vi "多影像平均_二值化_抓邊 _圓ROI.vi"() -> ()   [LabVIEW 2015]
uses:
  <vilib>/vision/Measure.llb/Edge Options.ctl
  <vilib>/vision/Measure.llb/Edge Polarity.ctl
  <vilib>/userdefined/High Color/IMAQdx.ctl
  <vilib>/Utility/miscctls.llb/LVPositionTypeDef.ctl
  <vilib>/Analysis/coordinate.llb/2D Cartesian Coordinate Rotation (Scalar).vi
  <vilib>/vision/NI_Vision_Development_Module.lvlib
  <vilib>/vision/driver/NI_Vision_Acquisition_Software.lvlib
  <resource>/objmgr/imaqdx.rc
  <vilib>/Analysis/NI_AALPro.lvlib
panel:
  in  "處理平均影像":bool
  out "Ellipse":T1 {"Minor Axis"."Point 2"."Y" format="%.2f"; "Minor Axis"."Point 2"."X" format="%.2f"; "Minor Axis"."Point 1"."Y" format="%.2f"; "Minor Axis"."Point 1"."X" format="%.2f"; "Major Axis"."Point 2"."Y" format="%.2f"; "Major Axis"."Point 2"."X" format="%.2f"; "Major Axis"."Point 1"."Y" format="%.2f"; "Major Axis"."Point 1"."X" format="%.2f"; "Center"."Y" format="%.2f"; "Center"."X" format="%.2f"}
  in  "載入影像":bool
  in  "拍攝影像":bool
  in  "影像數量":i32=4
  out "二值化影像陣列":T2[](array[plugin-control])
  out "全部影像Histograph":T3(graph)
  out "Image binary":T2(plugin-control)
  out "平均影像Histograph":T4(graph)
  out "Standard Deviation":sgl format="%#.2f"
  out "Mean":sgl format="%#.2f"
  out "影像陣列":T2[](array[plugin-control])
  in  "stop":bool
  in  "Horizontal Progress Bar":u8(slide) scale=0.0..255.0
  out "Image mean":T2(plugin-control)
  out "取像編號":i32
  out "取像視窗":T2(plugin-control)
  in  "Session In":T5="cam1"
  out "degrees":sgl
  in  "Edge Options":T6={"Edge Polarity"=0, "Kernel Size"=3, "Width"=3, "Minimum Edge Strength"=10.0, "Interpolation Type"=enum."Bilinear Fixed", "Data Processing Method"=enum."Average"} {"Edge Polarity" items=["All Edges", "Rising Edges", "Falling Edges"]; "Minimum Edge Strength" format="%.2f"; "Width" step=2; "Kernel Size" step=2}
  out "Gradient Information":dbl[][](graph)
  out "Line Segment":T8 {"Point 2"."Y" format="%.2f"; "Point 2"."X" format="%.2f"; "Point 1"."Y" format="%.2f"; "Point 1"."X" format="%.2f"}
  out "error out":errorcluster
  in  "Direction":T9(ring)
  in  "Process":T10(ring)
  out "Line Profile":T11(graph)
  in  "Gap":i32=10 min=1 max=300
  out "Image":T2(plugin-control)
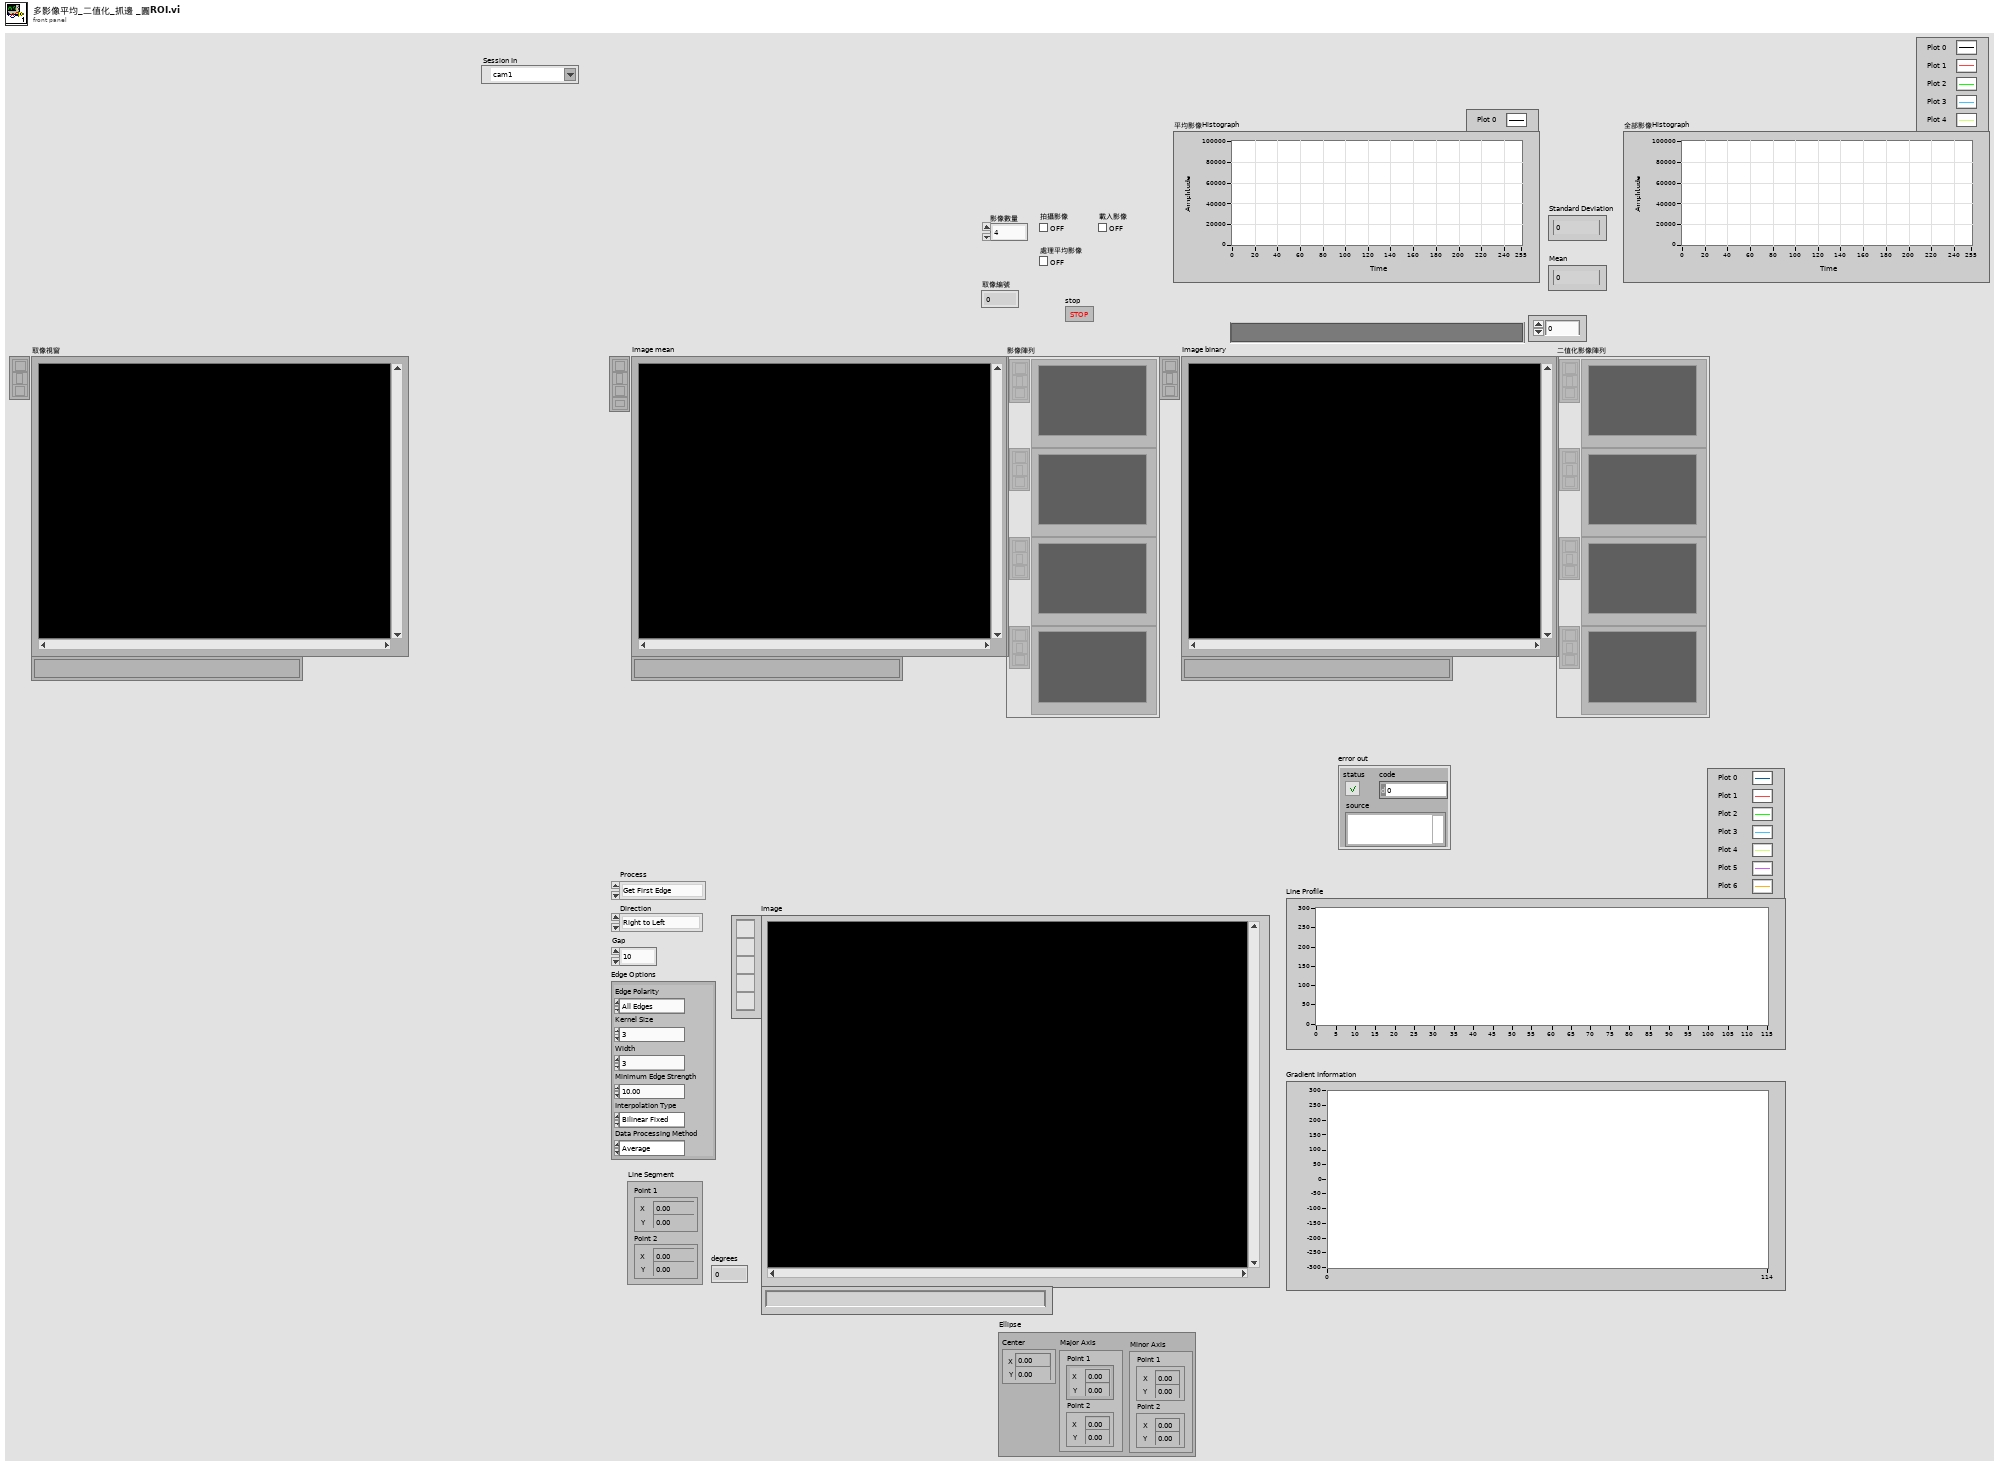
[diagram p1: front panel]
types:
  T1 = cluster{"Center":cluster{"X":sgl, "Y":sgl}, "Major Axis":cluster{"Point 1":cluster{"X":sgl, "Y":sgl}, "Point 2":cluster{"X":sgl, "Y":sgl}}, "Minor Axis":cluster{"Point 1":cluster{"X":sgl, "Y":sgl}, "Point 2":cluster{"X":sgl, "Y":sgl}}}
  T2 = typedef "IMAQ Image.ctl" = refnum<image>
  T3 = cluster{"Starting Value":sgl, "Incremental Value":sgl, "Histogram":u32[]}[]
  T4 = cluster{"Starting Value":sgl, "Incremental Value":sgl, "Histogram":u32[]}
  T5 = typedef "IMAQdx.ctl" = refnum<k21>
  T6 = typedef "Edge Options.ctl" = cluster{"Edge Polarity":T7, "Kernel Size":u32, "Width":u32, "Minimum Edge Strength":sgl, "Interpolation Type":enum32{"Zero Order", "Bilinear", "Quadratic", "Cubic", "Bilinear Fixed"}, "Data Processing Method":enum32{"Average", "Median"}}
  T7 = typedef "Edge Polarity.ctl" = u32
  T8 = cluster{"Point 1":cluster{"X":sgl, "Y":sgl}, "Point 2":cluster{"X":sgl, "Y":sgl}}
  T9 = enum16{"Right to Left", "Left  to Right", "Up to Down", "Down to Up", "Inner to Outer", "Outer to Inner"}
  T10 = enum16{"Get First Edge", "Get First + Last Edge", "Get All Edges", "Get Best Edge"}
  T11 = cluster{"x0":sgl, "dx":sgl, "Pixels Line":sgl[]}[]
  T12 = typedef "LVPositionTypeDef.ctl" = cluster{"Left":i32, "Top":i32}
  T13 = typedef "Image Type" = u32
  T14 = cluster{"Global Rectangle":i32[], "Contours":cluster{"Contour Type":u32, "ROI Type":u32, "Points":i32[]}[]}
  T15 = typedef "IMAQ Rectangle" = cluster{"Left":i32, "Top":i32, "Right":i32, "Bottom":i32, "Rotation":dbl}
  T16 = typedef "IMAQ Point" = cluster{"X":sgl, "Y":sgl}
  T17 = typedef "IMAQ Circle" = cluster{"Center X":i32, "Center Y":i32, "Inner Radius":i32, "Outer Radius":i32, "Start Angle":dbl, "End Angle":dbl}
  T18 = cluster{"Point 1":cluster{"x":dbl, "y":dbl}, "Point 2":cluster{"x":dbl, "y":dbl}}
  T19 = typedef "IMAQ Line" = cluster{"Start X":i32, "Start Y":i32, "End X":i32, "End Y":i32}
  T20 = cluster{"Contour Type":u32, "ROI Type":u32, "Points":i32[]}[]
  T21 = cluster{"Contour Type":u32, "ROI Type":u32, "Points":i32[]}
  T22 = typedef "ROI Descriptor" = cluster{"Global Rectangle":i32[], "Contours":cluster{"ID":enum32{"External", "Internal"}, "Type":u32, "Coordinates":i32[]}[]}
  T23 = typedef "Edge New.ctl" = cluster{"Location (Pixel)":cluster{"X":sgl, "Y":sgl}, "Location (Real-World)":cluster{"X":sgl, "Y":sgl}, "Distance (Pixel)":dbl, "Distance (Real-World)":dbl, "Strength":dbl, "Noise":dbl, "Rising?":bool}
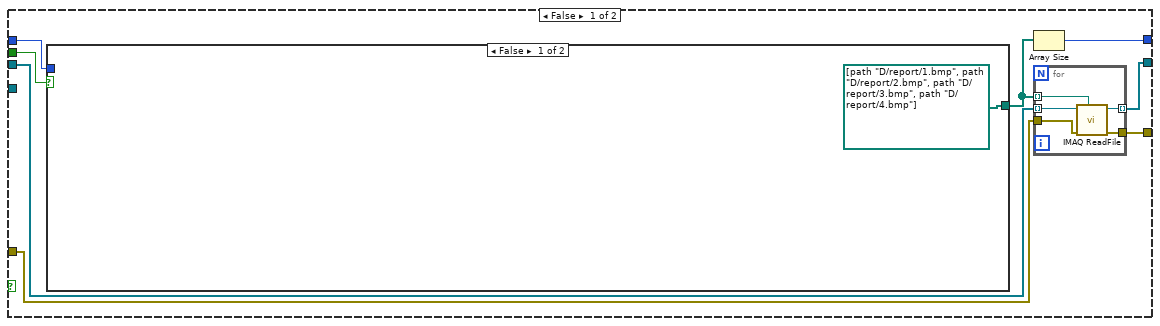
[diagram p2: hidden frame]
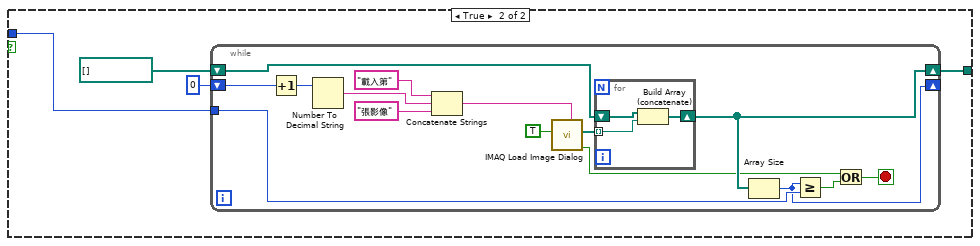
[diagram p3: hidden frame]
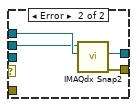
[diagram p4: hidden frame]
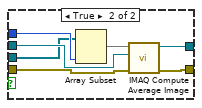
[diagram p5: hidden frame]
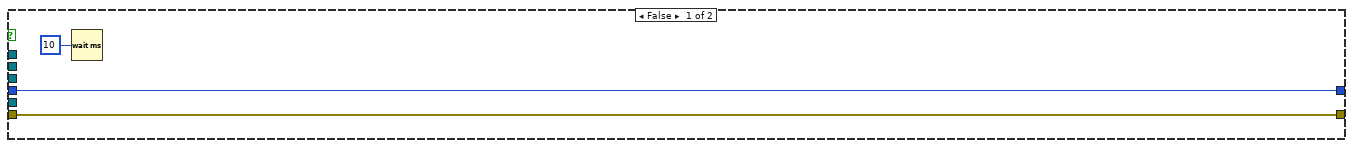
[diagram p6: hidden frame]
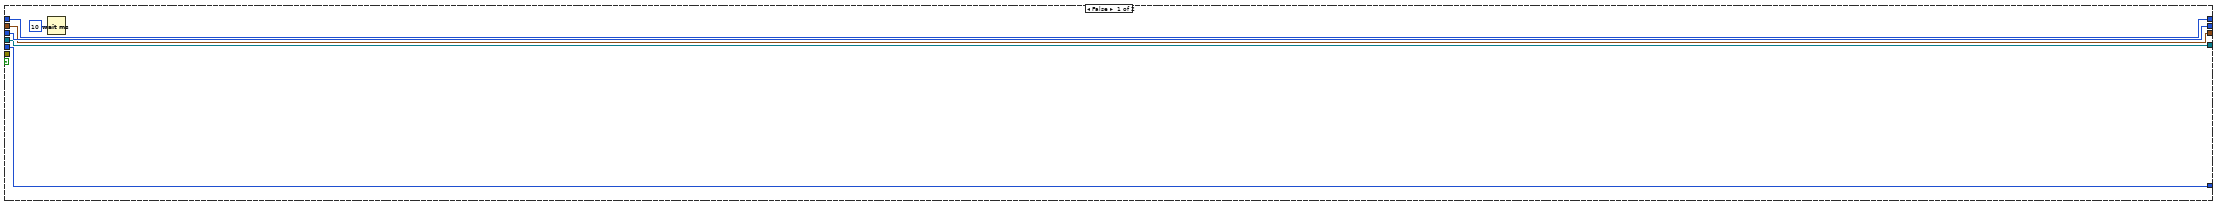
[diagram p7: hidden frame]
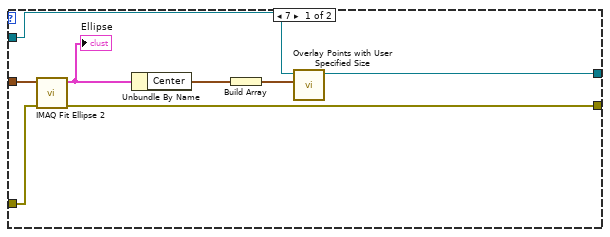
[diagram p8: hidden frame]
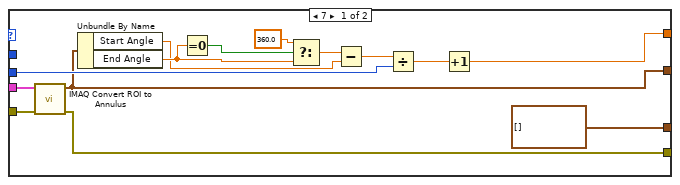
[diagram p9: hidden frame]
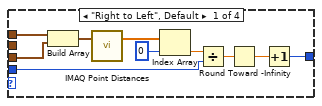
[diagram p10: hidden frame]
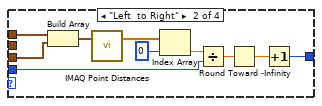
[diagram p11: hidden frame]
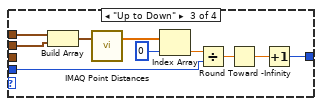
[diagram p12: hidden frame]
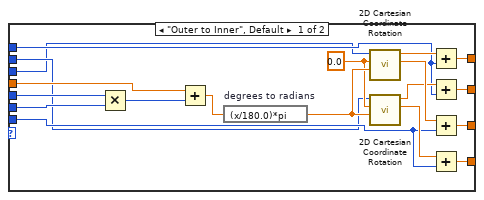
[diagram p14: hidden frame]
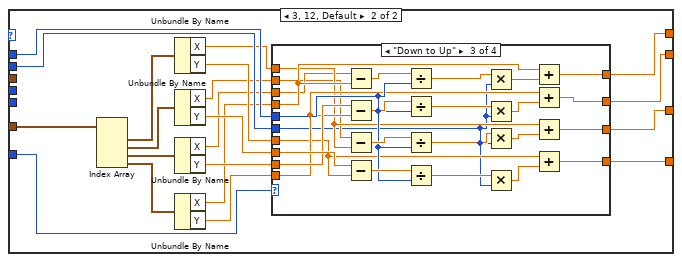
[diagram p15: hidden frame]
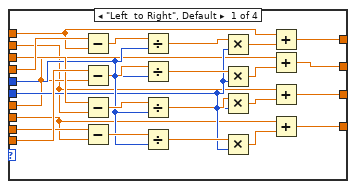
[diagram p16: hidden frame]
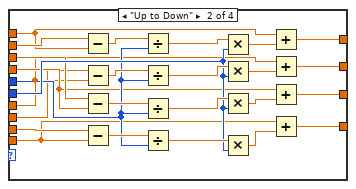
[diagram p17: hidden frame]
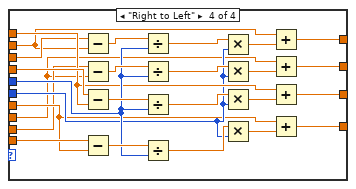
[diagram p18: hidden frame]
diagram:
  w40 = T13 0 items=["Grayscale (U8)", "Grayscale (I16)", "Grayscale (SGL)", "Complex (CSG)", "RGB (U32)", "HSL (U32)", "RGB (U64)", "Grayscale (U16)"] ("Image Type")
  w42 = i32[] [2] items=["No  event", "Click event", "Draw event", "Move event", "Size event", "Scroll event", "Activate event", "Close event", "Double click event"] ("Events list (all)")
  n1 = property on="Pane" class="Pane"("Origin"=T12 {"Left"=0, "Top"=0} ("Position")) -> (error out=w5:errorcluster)  [unwired: 2 in, 1 out]
  n2 = property on="Image" class="ImageControl"("ROI"=T14 {"Global Rectangle"=[450, 180, 600, 400], "Contours"=[{"Contour Type"=0, "ROI Type"=3, "Points"=[450, 180, 600, 400]}]}) -> ()  [unwired: 2 in, 2 out]
  n3 = flat-sequence {
    tunnel: [w68] -> w38
    tunnel: [w67] -> w37
    tunnel: [w65] -> w36
    tunnel: "影像數量" -> [w61]
    tunnel: [w63] -> w35
    tunnel: "拍攝影像" -> [w63]
    tunnel: [w62] -> w34
    tunnel: "載入影像" -> [w62]
    tunnel: [w61] -> w33
    tunnel: [w60] -> w32
    tunnel: [w57] -> w31
    tunnel: [w55] -> w30
    tunnel: [w53] -> w29
    tunnel: [w46] -> w28
    tunnel: w5 -> [w45]
    tunnel: w38 -> [w103]
    tunnel: w37 -> [w104]
    tunnel: [w102] -> w27
    tunnel: w36 -> [w101]
    tunnel: [w101] -> w26
    tunnel: w35 -> [w100]
    tunnel: w34 -> [w99]
    tunnel: w33 -> [w98]
    tunnel: [w97] -> w25
    tunnel: [w96] -> w24
    tunnel: w32 -> [w95]
    tunnel: [w95] -> w23
    tunnel: [w94] -> w22
    tunnel: w31 -> [w94]
    tunnel: w30 -> [w93]
    tunnel: [w93] -> w21
    tunnel: [w92] -> w20
    tunnel: w29 -> [w92]
    tunnel: w28 -> [w91]
    tunnel: w27 -> [w177]
    tunnel: w26 -> [w182]
    tunnel: w25 -> [w181]
    tunnel: w24 -> [w174]
    tunnel: w23 -> [w180]
    tunnel: [w180] -> w19
    tunnel: [w171] -> w18
    tunnel: [w177] -> w17
    tunnel: [w176] -> w16
    tunnel: [w179] -> w15
    tunnel: w22 -> [w179]
    tunnel: w21 -> [w175]
    tunnel: [w175] -> w14
    tunnel: [w178] -> w13
    tunnel: w20 -> [w178]
    tunnel: w19 -> [w202]
    tunnel: w18 -> [w197]
    tunnel: w17 -> [w203]
    tunnel: w16 -> [w195]
    tunnel: w15 -> [w201]
    tunnel: w14 -> [w196]
    tunnel: w13 -> [w198]
    tunnel: [w195] -> w9
    tunnel: [w194] -> w4
    frame #0 {
      w59 = T13 0 items=["Grayscale (U8)", "Grayscale (I16)", "Grayscale (SGL)", "Complex (CSG)", "RGB (U32)", "HSL (U32)", "RGB (U64)", "Grayscale (U16)"] ("Image Type")
      w52 = 20
      w64 = T13 0 items=["Grayscale (U8)", "Grayscale (I16)", "Grayscale (SGL)", "Complex (CSG)", "RGB (U32)", "HSL (U32)", "RGB (U64)", "Grayscale (U16)"] ("Image Type")
      n4 = call <vilib>:"IMAQdx Open Camera.vi"("error in"=w45, "Session In"="Session In") -> ("error out"=w54:errorcluster, "Session Out"=w68:T5)  [unwired: 8 in]
      n5 = for {
        N: w52 -> [_]
        tunnel: [w90] -> w67 mode=indexing
        tunnel: w54 -> [w89]
        tunnel: [w88] -> w51
        i -> [w87]
        n6 = Number To Decimal String(number=w87) -> (decimal integer string=w85:string)  [unwired: 1 in]
        n7 = Concatenate Strings("Image", w85) -> (w84:string)
        n8 = call "IMAQ Create"("Image Name"=w84, "error in (no error)"=w89) -> ("New Image"=w90:T2, "error out"=w88:errorcluster)  [unwired: 3 in]
      }
      n9 = for {
        N: w52 -> [_]
        tunnel: [w76] -> w53 mode=indexing
        tunnel: w51 -> [w75]
        tunnel: [w70] -> _
        tunnel: [w70] -> w50 mode=indexing
        i -> [w74]
        n10 = Number To Decimal String(number=w74) -> (decimal integer string=w72:string)  [unwired: 1 in]
        n11 = Concatenate Strings("Histogram Mask", w72) -> (w71:string)
        n12 = call "IMAQ Create"("Image Name"=w71, "error in (no error)"=w75) -> ("New Image"=w76:T2, "error out"=w70:errorcluster)  [unwired: 3 in]
      }
      n13 = for {
        N: w52 -> [_]
        tunnel: [w83] -> w60 mode=indexing
        tunnel: w50 -> [w82] mode=indexing
        tunnel: [w81] -> w47
        i -> [w80]
        n14 = Number To Decimal String(number=w80) -> (decimal integer string=w78:string)  [unwired: 1 in]
        n15 = Concatenate Strings("Threshole", w78) -> (w77:string)
        n16 = call "IMAQ Create"("Image Name"=w77, "error in (no error)"=w82) -> ("New Image"=w83:T2, "error out"=w81:errorcluster)  [unwired: 3 in]
      }
      n17 = call "IMAQ Create"("Image Name"="imageMeans", "Image Type"=w64, "error in (no error)"=w47) -> ("New Image"=w65:T2, "error out"=w49:errorcluster)  [unwired: 2 in]
      n18 = call "IMAQ Create"("Image Name"="Histogram Mask", "error in (no error)"=w49) -> ("New Image"=w55:T2, "error out"=w48:errorcluster)  [unwired: 3 in]
      n19 = call "IMAQ Create"("Image Name"="imageBinary", "Image Type"=w59, "error in (no error)"=w48) -> ("New Image"=w57:T2, "error out"=w46:errorcluster)  [unwired: 2 in]
    }
    frame #1 {
      n20 = case shown="True" w100 {
        tunnel: w104 -> [w109 w148]
        tunnel: w103 -> [_ w147]
        tunnel: w91 -> [w108 w145]
        tunnel: [w110 w144] -> w102
        tunnel: w99 -> [w112 _]
        tunnel: w98 -> [w111 w142]
        tunnel: [w107 w143] -> w97
        tunnel: [w105 w142] -> w96
        frame False {
          n21 = case shown="False" w112 {
            tunnel: [path[] [path "D:/report/1.bmp", path "D:/report/2.bmp", path "D:/report/3.bmp", path "D:/report/4.bmp"] w117] -> w106
            tunnel: w111 -> [_ w116]
            frame False {
            }
            frame True {
              n22 = while {
                tunnel: w116 -> [w129]
                shift-right: [w132] -> w117
                shift-left: path[] [] -> [w128]
                shift-right: [w127] -> _
                shift-left: 0 -> [w126]
                stop <- w119 stop-if-true
                n23 = Increment(x=w126) -> (x+1=w125:i32)
                n24 = Number To Decimal String(number=w125) -> (decimal integer string=w122:string)  [unwired: 1 in]
                n25 = Concatenate Strings("載入第", w122, "張影像") -> (w121:string)
                n26 = call "IMAQ Load Image Dialog"("Button Label"=w121, "Multiple Files? (No)"=TRUE) -> ("Cancelled?"=w120:bool, "Paths"=w130:path[])  [unwired: 7 in, 1 out]
                n27 = for {
                  tunnel: w130 -> [w134] mode=indexing
                  shift-right: [w133] -> w132
                  shift-left: w128 -> [w135]
                  n28 = Build Array (concatenate)(w135, w134) -> (w133:path[])
                }
                n29 = Array Size(array=w132) -> (size(s)=w127:i32)
                n30 = Greater Or Equal?(x=w127, y=w129) -> (x >= y?=w118:bool)
                n31 = Or(x=w120, y=w118) -> (x .or. y?=w119:bool)
              }
            }
          }
          n32 = Array Size(array=w106) -> (size(s)=w105:i32)
          n33 = for {
            tunnel: w106 -> [w140] mode=indexing
            tunnel: [w139] -> w110 mode=indexing
            tunnel: w109 -> [w138] mode=indexing
            tunnel: w108 -> [w137]
            tunnel: [w136] -> w107
            n34 = call "IMAQ ReadFile"("File Path"=w140, "error in (no error)"=w137, "Image"=w138) -> ("error out"=w136:errorcluster, "Image Out"=w139:T2)  [unwired: 4 in, 3 out]
          }
        }
        frame True {
          n35 = property on="Pane" class="Pane"("Origin"=T12 {"Left"=-951, "Top"=0} ("Position")) -> ()  [unwired: 2 in, 2 out]
          n36 = for {
            N: w142 -> [_]
            tunnel: w148 -> [w151] mode=indexing
            tunnel: w147 -> [w149]
            tunnel: dbl[] [0.01, 0.03, 0.05, 0.07] -> [w159] mode=indexing
            tunnel: w145 -> [w154]
            tunnel: [w158] -> w144 mode=indexing
            tunnel: [w156] -> w143
            i -> [w160]
            w157 = T13 0 items=["Grayscale (U8)", "Grayscale (I16)", "Grayscale (SGL)", "Complex (CSG)", "RGB (U32)", "HSL (U32)", "RGB (U64)", "Grayscale (U16)"] ("Image Type")
            n37 = property class="IMAQdx"(reference=w149, error in=w154, "ActiveAttribute"="CameraAttributes::Exposure::Value", "ValueDBL"=w159) -> (reference out=w150:T5, error out=w152:errorcluster)
            n38 = case shown="No Error" w152 {
              tunnel: [w165 w169] -> w156
              tunnel: [w164 w166] -> w155
              tunnel: w152 -> [w163 _]
              tunnel: w150 -> [w162 _]
              tunnel: w151 -> [w161 w168]
              tunnel: w149 -> [_ w167]
              frame No Error {
                n39 = call <vilib>:"IMAQdx Snap2.vi"("error in"=w163, "Image In"=w161, "Session In"=w162) -> ("error out"=w165:errorcluster, "Image Out"=w164:T2)  [unwired: 6 in, 1 out]
              }
              frame Error {
                n40 = call <vilib>:"IMAQdx Snap2.vi"("Image In"=w168, "Session In"=w167) -> ("error out"=w169:errorcluster, "Image Out"=w166:T2)  [unwired: 7 in, 1 out]
              }
            }
            "取像視窗" <- w155
            n41 = call "IMAQ Cast Image"("Image Type"=w157, "Image Src"=w155) -> ("Image Dst Out"=w158:T2)  [unwired: 8 in, 1 out]
            "取像編號" <- w160
          }
        }
      }
    }
    frame #2 {
      n42 = Not Equal?(x=w174, y=1) -> (x != y?=w172:bool)
      n43 = property on="Pane" class="Pane"("Origin"=T12 {"Left"=0, "Top"=0} ("Position")) -> ()  [unwired: 2 in, 2 out]
      n44 = case shown="False" w172 {
        tunnel: w182 -> [_ w193]
        tunnel: w181 -> [w186 w192]
        tunnel: w174 -> [_ w191]
        tunnel: [w186 w189] -> w171
        tunnel: w177 -> [w184 w188]
        tunnel: [w183 w187] -> w176
        frame False {
          n45 = Index Array(array=w184, index=0) -> (element=w183:T2)
        }
        frame True {
          n46 = Array Subset(array=w188, length=w191) -> (w190:T2[])  [unwired: 1 in]
          n47 = call "IMAQ Compute Average Image"("error in (no error)"=w192, "Image Dst"=w193, "Images"=w190) -> ("error out"=w189:errorcluster, "Image Dst Out"=w187:T2)  [unwired: 7 in]
        }
      }
      "Image mean" <- w176
    }
    frame #3 {
      w199 = i32[] [2] items=["No  event", "Click event", "Draw event", "Move event", "Size event", "Scroll event", "Activate event", "Close event", "Double click event"] ("Events list (all)")
      n48 = property on="Image mean" class="ImageControl"("ROI"=T14 {"Global Rectangle"=[0, 0, 1292, 964], "Contours"=[{"Contour Type"=0, "ROI Type"=3, "Points"=[0, 0, 1292, 964]}]}) -> ()  [unwired: 2 in, 2 out]
      n49 = while {
        tunnel: w203 -> [w225]
        tunnel: w202 -> [w224]
        tunnel: w195 -> [w222]
        tunnel: w196 -> [w223]
        tunnel: w201 -> [w221]
        tunnel: w199 -> [w220]
        shift-right: [w217] -> _
        shift-left: _ -> [w215]
        tunnel: w198 -> [w210]
        tunnel: w197 -> [w209]
        tunnel: [w207] -> w194
        i -> [w218]
        stop <- w204 stop-if-true
        n50 = invoke on="Image mean" class="ImageControl" method="Get Last Event"("Which Events"=w220) -> ("Type"=w219:i32)  [unwired: 7 in, 7 out]
        n51 = property on="平均影像Histograph" class="WFGraph (strict)"() -> ("YScale.Maximum"=w208:dbl)  [unwired: 2 in, 2 out]
        n52 = Or(x="stop", y="處理平均影像") -> (x .or. y?=w204:bool)
        n53 = property on="全部影像Histograph" class="WFGraph (strict)"("YScale.Maximum"=w208) -> ()  [unwired: 2 in, 2 out]
        n54 = Not Equal?(x="Horizontal Progress Bar", y=w215) -> (x != y?=w212:bool)
        n55 = Not Equal To 0?(x=w219) -> (x != 0?=w213:bool)
        n56 = Equal To 0?(x=w218) -> (x = 0?=w214:bool)
        n57 = Compound Arithmetic op=OR(w214, w213, w212) -> (w211:bool)
        n58 = case shown="True" w211 {
          tunnel: w225 -> [_ w234]
          tunnel: w224 -> [_ w262]
          tunnel: w223 -> [_ w231]
          tunnel: w222 -> [_ w232]
          tunnel: w221 -> [_ w249]
          tunnel: "Horizontal Progress Bar" -> [w227 w247]
          tunnel: [w227 w247] -> w217
          tunnel: w210 -> [_ w245]
          tunnel: w209 -> [w226 w236]
          tunnel: [w226 w229] -> w207
          frame False {
            n59 = Wait (ms)(milliseconds to wait=u32 10) -> ()  [unwired: 1 out]
          }
          frame True {
            n60 = property on="Image mean" class="ImageControl"() -> ("ROI"=w244:T14)  [unwired: 2 in, 2 out]
            n61 = property on="Image binary" class="ImageControl"("Zoom to Fit Mode"=TRUE) -> ()  [unwired: 2 in, 2 out]
            n62 = call "IMAQ Convert ROI to Rectangle"("error in (no error)"=w236, "ROI Descriptor"=w244) -> ("error out"=w237:errorcluster, "Rectangle"=w254:T15)  [unwired: 7 in]
            n63 = Unbundle By Name(w254) -> ("Left"=w250:i32, "Top"=w251:i32, "Right"=w252:i32, "Bottom"=w253:i32)
            n64 = Build Array(w250, w251, w252, w253) -> (w243:i32[])
            n65 = for {
              tunnel: w234 -> [w265] mode=indexing
              tunnel: w262 -> [w279] mode=indexing
              tunnel: [w278] -> w261 mode=indexing
              tunnel: [w266] -> w257 mode=indexing
              tunnel: w247 -> [w275]
              tunnel: w245 -> [w272] mode=indexing
              tunnel: w244 -> [w274]
              tunnel: w243 -> [w273]
              tunnel: [w269] -> w238
              tunnel: w237 -> [w268]
              tunnel: [w267] -> w233 mode=indexing
              n66 = call "IMAQ ROIToMask"("error in (no error)"=w268, "ROI Descriptor"=w274, "Image"=w272, "Image Model"=w265) -> ("error out"=w271:errorcluster, "Image Out"=w264:T2)  [unwired: 2 in, 1 out]
              n67 = call "IMAQ Extract 2"("Optional Rectangle"=w273, "error in (no error)"=w271, "Image Dst"=w272, "Image Src"=w265) -> ("error out"=w270:errorcluster, "Image Dst Out"=w267:T2)  [unwired: 6 in]
              n68 = Bundle By Name(cluster=cluster{"Lower value":sgl, "Upper value":sgl} {"Lower value"=128.0, "Upper value"=255.0} ("Range"), "Lower value"=w275) -> (w276:cluster{"Lower value":sgl, "Upper value":sgl})
              n69 = call "IMAQ Histograph"("error in (no error)"=w270, "Image"=w264) -> ("error out"=w263:errorcluster, "Histogram Graph"=w266:T4)  [unwired: 6 in, 2 out]
              n70 = call "IMAQ Threshold"("error in (no error)"=w263, "Range"=w276, "Image Dst"=w279, "Image Src"=w267) -> ("error out"=w269:errorcluster, "Image Dst Out"=w278:T2)  [unwired: 6 in]
            }
            "二值化影像陣列" <- w261
            "影像陣列" <- w233
            n71 = call "IMAQ ROIToMask"("error in (no error)"=w238, "ROI Descriptor"=w244, "Image"=w231, "Image Model"=w232) -> ("error out"=w241:errorcluster, "Image Out"=w230:T2)  [unwired: 2 in, 1 out]
            n72 = call "IMAQ Extract 2"("Optional Rectangle"=w243, "error in (no error)"=w241, "Image Dst"=w231, "Image Src"=w232) -> ("error out"=w240:errorcluster, "Image Dst Out"=w242:T2)  [unwired: 6 in]
            n73 = call "IMAQ Histograph"("error in (no error)"=w240, "Image"=w230) -> ("error out"=w239:errorcluster, "Standard  Deviation"=→"Standard Deviation":sgl, "Mean Value"=→"Mean":sgl, "Histogram Graph"=w255:T4)  [unwired: 6 in]
            "平均影像Histograph" <- w255
            n74 = Bundle By Name(cluster=cluster{"Lower value":sgl, "Upper value":sgl} {"Lower value"=128.0, "Upper value"=255.0} ("Range"), "Lower value"=w247) -> (w260:cluster{"Lower value":sgl, "Upper value":sgl})
            n75 = Build Array (concatenate)(w255, w257) -> (→"全部影像Histograph":T3)
            n76 = call "IMAQ Threshold"("error in (no error)"=w239, "Range"=w260, "Image Dst"=w249, "Image Src"=w242) -> ("error out"=w229:errorcluster, "Image Dst Out"=→"Image binary":T2)  [unwired: 6 in]
          }
        }
      }
    }
  }
  n77 = property on="Pane" class="Pane"(error in=w4, "Origin"=T12 {"Left"=0, "Top"=1000} ("Position")) -> (error out=w3:errorcluster)  [unwired: 1 in, 1 out]
  n78 = call "IMAQ Create"("Image Name"="Edge Detection Source", "error in (no error)"=w3) -> ("New Image"=w7:T2, "error out"=w6:errorcluster)  [unwired: 3 in]
  n79 = call "IMAQ Copy"("Image Dst"=w7, "Image Src"=w9) -> ("Image Dst Out"=w8:T2)  [unwired: 4 in, 1 out]
  n80 = call "IMAQ Cast Image"("Image Type"=w40, "error in (no error)"=w6, "Image Src"=w8) -> ("error out"=w39:errorcluster, "Image Dst Out"=w41:T2)  [unwired: 7 in]
  n81 = while {
    tunnel: w39 -> [w284]
    tunnel: w41 -> [w302]
    tunnel: w42 -> [w286]
    shift-right: [w301] -> _
    shift-left: _ -> [w300]
    shift-right: [w293] -> _
    shift-left: _ -> [w294]
    shift-right: [w288] -> _
    shift-left: _ -> [w289]
    shift-right: [w282] -> _
    shift-left: _ -> [w281]
    stop <- FALSE stop-if-true
    n82 = invoke on="Image" class="ImageControl" method="Get Last Event"("Which Events"=w286) -> ("Type"=w285:i32)  [unwired: 7 in, 7 out]
    n83 = Not Equal?(x=w300, y="Direction") -> (x != y?=w299:bool)
    n84 = Not Equal To 0?(x=w285) -> (x != 0?=w298:bool)
    n85 = Not Equal?(x=w294, y="Gap") -> (x != y?=w292:bool)
    n86 = Not Equal?(x=w289, y="Edge Options") -> (x != y?=w287:bool)
    n87 = Not Equal?(x=w281, y="Process") -> (x != y?=w280:bool)
    n88 = Compound Arithmetic op=OR(w299, w298, w292, w287, w280) -> (w297:bool)
    n89 = case shown="True" w297 {
      tunnel: w302 -> [w306 w338]
      tunnel: w284 -> [_ w312]
      tunnel: "Direction" -> [w308 w334]
      tunnel: [w308 w334] -> w301
      tunnel: "Gap" -> [w307 w326]
      tunnel: [w307 w326] -> w293
      tunnel: [w306 w320] -> w291
      tunnel: "Edge Options" -> [w305 w330]
      tunnel: [w305 w330] -> w288
      tunnel: "Process" -> [w304 w310]
      tunnel: [w304 w310] -> w282
      frame False {
        n90 = Wait (ms)(milliseconds to wait=u32 10) -> ()  [unwired: 1 out]
      }
      frame True {
        n91 = property on="Gradient Information" class="WFChart (strict)"(error in=w312, "History Data"=dbl[][] []) -> (error out=w311:errorcluster)  [unwired: 1 in, 1 out]
        n92 = property on="Image" class="ImageControl"() -> ("ROI"=w318:T14)  [unwired: 2 in, 2 out]
        n93 = Unbundle By Name(w318) -> ("Contours"=w325:T20)
        n94 = Index Array(array=w325, index=0) -> (element=w323:T21)
        n95 = Unbundle By Name(w323) -> ("ROI Type"=w319:u32)
        n96 = call "IMAQ Clear Overlay"("error in (no error)"=w311, "Image"=w338) -> ("error out"=w337:errorcluster, "Image Out"=w332:T2)  [unwired: 8 in]
        n97 = case shown="3, 12, Default" w319 {
          tunnel: w318 -> [w369 w384]
          tunnel: w337 -> [w371 w392]
          tunnel: w334 -> [_ w391]
          tunnel: w326 -> [w372 w390]
          tunnel: [w374 w387] -> w333
          tunnel: [w370 w385] -> w331
          tunnel: [T16[] [] ("Rectangle Points") w383] -> w316
          tunnel: [w367 T17 {"Center X"=0, "Center Y"=0, "Inner Radius"=0, "Outer Radius"=0, "Start Angle"=0.0, "End Angle"=0.0} ("Annulus")] -> w317
          frame 7 {
            n98 = call "IMAQ Convert ROI to Annulus"("error in (no error)"=w371, "ROI Descriptor"=w369) -> ("error out"=w370:errorcluster, "Annulus"=w367:T17)  [unwired: 7 in]
            n99 = Unbundle By Name(w367) -> ("Start Angle"=w373:dbl, "End Angle"=w375:dbl)
            n100 = Equal To 0?(x=w375) -> (x = 0?=w380:bool)
            n101 = Select(t=360.0, s=w380, f=w375) -> (s? t:f=w378:dbl)
            n102 = Subtract(x=w378, y=w373) -> (x-y=w377:dbl)
            n103 = Divide(x=w377, y=w372) -> (x/y=w376:dbl)
            n104 = Increment(x=w376) -> (x+1=w374:dbl)
          }
          frame 3, 12, Default {
            n105 = call "IMAQ Convert ROI to Rectangle"("error in (no error)"=w392, "ROI Descriptor"=w384) -> ("error out"=w385:errorcluster, "Rectangle"=w381:T15)  [unwired: 7 in]
            n106 = call "IMAQ Convert Rectangle to ROI (Polygon)"("Rectangle"=w381) -> ("Rectangle Points"=w383:T16[])  [unwired: 7 in, 2 out]
            n107 = Index Array(array=w383) -> (element #1=w389:T16, element #2=w388:T16, element #4=w386:T16)  [unwired: 4 in, 1 out]
            n108 = case shown="\"Down to Up\"" w391 {
              tunnel: w390 -> [w400 w410 w420 w430]
              tunnel: [w399 w409 w419 w429] -> w387
              tunnel: w389 -> [w396 w406 w418 w426]
              tunnel: w386 -> [w395 w405 _ _]
              tunnel: w388 -> [_ _ w414 w425]
              frame "Right to Left", Default {
                n109 = Build Array(w396, w395) -> (w398:T16[])
                n110 = call "IMAQ Point Distances"("Points"=w398) -> ("Distances"=w397:sgl[])  [unwired: 4 in, 1 out]
                n111 = Index Array(array=w397, index=0) -> (element=w393:sgl)
                n112 = Divide(x=w393, y=w400) -> (x/y=w401:sgl)
                n113 = Round Toward -Infinity(1:w401) -> (0:w402:sgl)
                n114 = Increment(x=w402) -> (x+1=w399:i32)
              }
              frame "Left  to Right" {
                n115 = Build Array(w406, w405) -> (w408:T16[])
                n116 = call "IMAQ Point Distances"("Points"=w408) -> ("Distances"=w407:sgl[])  [unwired: 4 in, 1 out]
                n117 = Index Array(array=w407, index=0) -> (element=w403:sgl)
                n118 = Divide(x=w403, y=w410) -> (x/y=w411:sgl)
                n119 = Round Toward -Infinity(1:w411) -> (0:w412:sgl)
                n120 = Increment(x=w412) -> (x+1=w409:i32)
              }
              frame "Up to Down" {
                n121 = Build Array(w418, w414) -> (w417:T16[])
                n122 = call "IMAQ Point Distances"("Points"=w417) -> ("Distances"=w416:sgl[])  [unwired: 4 in, 1 out]
                n123 = Index Array(array=w416, index=0) -> (element=w415:sgl)
                n124 = Divide(x=w415, y=w420) -> (x/y=w421:sgl)
                n125 = Round Toward -Infinity(1:w421) -> (0:w422:sgl)
                n126 = Increment(x=w422) -> (x+1=w419:i32)
              }
              frame "Down to Up" {
                n127 = Build Array(w426, w425) -> (w428:T16[])
                n128 = call "IMAQ Point Distances"("Points"=w428) -> ("Distances"=w427:sgl[])  [unwired: 4 in, 1 out]
                n129 = Index Array(array=w427, index=0) -> (element=w424:sgl)
                n130 = Divide(x=w424, y=w430) -> (x/y=w431:sgl)
                n131 = Round Toward -Infinity(1:w431) -> (0:w432:sgl)
                n132 = Increment(x=w432) -> (x+1=w429:i32)
              }
            }
          }
        }
        n133 = for {
          N: w333 -> [w475]
          tunnel: w334 -> [w469]
          tunnel: [w484] -> w327
          tunnel: w332 -> [w470]
          tunnel: w331 -> [w467]
          tunnel: [w483] -> w321
          tunnel: w310 -> [w485]
          tunnel: w330 -> [w482]
          tunnel: [w481] -> w329 mode=indexing
          tunnel: [w480] -> w335 mode=indexing
          tunnel: [w479] -> w328 mode=indexing
          tunnel: w319 -> [w466]
          tunnel: w326 -> [w465]
          tunnel: w317 -> [w463]
          tunnel: w316 -> [w462]
          i -> [w464]
          w474 = 1
          w459 = cluster{"X":i32, "Y":i32} {"X"=0, "Y"=0} ("Start Point")
          n134 = Equal?(x=w464, y=w474) -> (x = y?=w472:bool)
          n135 = Subtract(x=w475, y=w474) -> (x-y=w473:i32)
          n136 = case shown="7" w466 {
            tunnel: [w502 w562] -> w451
            tunnel: [w499 w561] -> w450
            tunnel: w464 -> [_ w560]
            tunnel: w475 -> [_ w559]
            tunnel: w469 -> [w498 w558]
            tunnel: [w501 w557] -> w449
            tunnel: [w500 w556] -> w448
            tunnel: w465 -> [w504 _]
            tunnel: w464 -> [w503 _]
            tunnel: w463 -> [w497 _]
            tunnel: w462 -> [_ w555]
            frame 7 {
              n137 = Unbundle By Name(w497) -> ("Center X"=w496:i32, "Center Y"=w495:i32, "Inner Radius"=w494:i32, "Outer Radius"=w493:i32, "Start Angle"=w492:dbl)  [unwired: 1 out]
              n138 = case shown="\"Inner to Outer\"" w498 {
                tunnel: w495 -> [w507 w542]
                tunnel: w494 -> [w506 w541]
                tunnel: w493 -> [w505 w540]
                tunnel: w492 -> [w510 w539]
                tunnel: w504 -> [w508 w538]
                tunnel: w503 -> [w509 w529]
                tunnel: [w515 w524] -> w502
                tunnel: [w513 w528] -> w501
                tunnel: w496 -> [w511 w527]
                tunnel: [w512 w526] -> w500
                tunnel: [w514 w525] -> w499
                frame "Outer to Inner", Default {
                  w518 = 0.0 ("y")
                  n139 = Multiply(x=w509, y=w508) -> (x*y=w517:i32)
                  n140 = Add(x=w510, y=w517) -> (x+y=w516:dbl)
                  n141 = expression code="(x/180.0)*pi" "degrees to radians"(w516) -> (w519:dbl)
                  n142 = call-poly <vilib>:"2D Cartesian Coordinate Rotation.vi"("theta"=w519, "y"=w518, "x"=w505) -> ("y out"=w522:dbl, "x out"=w523:dbl)  [unwired: 6 in, 1 out]
                  n143 = call-poly <vilib>:"2D Cartesian Coordinate Rotation.vi"("theta"=w519, "y"=w518, "x"=w506) -> ("y out"=w521:dbl, "x out"=w520:dbl)  [unwired: 6 in, 1 out]
                  n144 = Add(x=w523, y=w511) -> (x+y=w515:dbl)
                  n145 = Add(x=w520, y=w511) -> (x+y=w512:dbl)
                  n146 = Add(x=w522, y=w507) -> (x+y=w514:dbl)
                  n147 = Add(x=w521, y=w507) -> (x+y=w513:dbl)
                }
                frame "Inner to Outer" {
                  w532 = 0.0 ("y")
                  n148 = Multiply(x=w529, y=w538) -> (x*y=w531:i32)
                  n149 = Add(x=w539, y=w531) -> (x+y=w530:dbl)
                  n150 = expression code="(x/180.0)*pi" "degrees to radians"(w530) -> (w533:dbl)
                  n151 = call-poly <vilib>:"2D Cartesian Coordinate Rotation.vi"("theta"=w533, "y"=w532, "x"=w541) -> ("y out"=w536:dbl, "x out"=w537:dbl)  [unwired: 6 in, 1 out]
                  n152 = call-poly <vilib>:"2D Cartesian Coordinate Rotation.vi"("theta"=w533, "y"=w532, "x"=w540) -> ("y out"=w535:dbl, "x out"=w534:dbl)  [unwired: 6 in, 1 out]
                  n153 = Add(x=w537, y=w527) -> (x+y=w524:dbl)
                  n154 = Add(x=w534, y=w527) -> (x+y=w526:dbl)
                  n155 = Add(x=w536, y=w542) -> (x+y=w525:dbl)
                  n156 = Add(x=w535, y=w542) -> (x+y=w528:dbl)
                }
              }
            }
            frame 3, 12, Default {
              n157 = Index Array(array=w555) -> (element #1=w554:T16, element #2=w553:T16, element #3=w552:T16, element #4=w551:T16)  [unwired: 4 in]
              n158 = Unbundle By Name(w554) -> ("X"=w550:sgl, "Y"=w549:sgl)
              n159 = Unbundle By Name(w553) -> ("X"=w548:sgl, "Y"=w547:sgl)
              n160 = Unbundle By Name(w552) -> ("X"=w546:sgl, "Y"=w545:sgl)
              n161 = Unbundle By Name(w551) -> ("X"=w544:sgl, "Y"=w543:sgl)
              n162 = case shown="\"Down to Up\"" w558 {
                tunnel: [w573 w592 w618 w643] -> w562
                tunnel: [w568 w591 w617 w644] -> w556
                tunnel: [w571 w589 w615 w641] -> w561
                tunnel: [w567 w590 w616 w642] -> w557
                tunnel: w544 -> [w586 w597 w623 w653]
                tunnel: w550 -> [w564 w599 w622 w652]
                tunnel: w559 -> [w577 w601 w628 w654]
                tunnel: w560 -> [w576 w602 w619 w651]
                tunnel: w543 -> [w583 w593 w625 w648]
                tunnel: w549 -> [w566 w595 w624 w647]
                tunnel: w546 -> [w580 w598 w621 w650]
                tunnel: w548 -> [w565 w600 w620 w649]
                tunnel: w545 -> [w575 w594 w626 w646]
                tunnel: w547 -> [w563 w596 w627 w645]
                frame "Left  to Right", Default {
                  n163 = Subtract(x=w586, y=w564) -> (x-y=w587:sgl)
                  n164 = Subtract(x=w583, y=w566) -> (x-y=w585:sgl)
                  n165 = Subtract(x=w580, y=w565) -> (x-y=w582:sgl)
                  n166 = Subtract(x=w575, y=w563) -> (x-y=w578:sgl)
                  n167 = Divide(x=w587, y=w577) -> (x/y=w588:sgl)
                  n168 = Divide(x=w585, y=w577) -> (x/y=w584:sgl)
                  n169 = Divide(x=w582, y=w577) -> (x/y=w581:sgl)
                  n170 = Divide(x=w578, y=w577) -> (x/y=w579:sgl)
                  n171 = Multiply(x=w588, y=w576) -> (x*y=w574:sgl)
                  n172 = Multiply(x=w584, y=w576) -> (x*y=w572:sgl)
                  n173 = Multiply(x=w581, y=w576) -> (x*y=w570:sgl)
                  n174 = Multiply(x=w579, y=w576) -> (x*y=w569:sgl)
                  n175 = Add(x=w564, y=w574) -> (x+y=w573:sgl)
                  n176 = Add(x=w566, y=w572) -> (x+y=w571:sgl)
                  n177 = Add(x=w565, y=w570) -> (x+y=w568:sgl)
                  n178 = Add(x=w563, y=w569) -> (x+y=w567:sgl)
                }
                frame "Up to Down" {
                  n179 = Subtract(x=w600, y=w599) -> (x-y=w613:sgl)
                  n180 = Subtract(x=w596, y=w595) -> (x-y=w612:sgl)
                  n181 = Subtract(x=w598, y=w597) -> (x-y=w610:sgl)
                  n182 = Subtract(x=w594, y=w593) -> (x-y=w607:sgl)
                  n183 = Divide(x=w613, y=w601) -> (x/y=w614:sgl)
                  n184 = Divide(x=w612, y=w601) -> (x/y=w611:sgl)
                  n185 = Divide(x=w610, y=w601) -> (x/y=w609:sgl)
                  n186 = Divide(x=w607, y=w601) -> (x/y=w608:sgl)
                  n187 = Multiply(x=w614, y=w602) -> (x*y=w606:sgl)
                  n188 = Multiply(x=w611, y=w602) -> (x*y=w605:sgl)
                  n189 = Multiply(x=w609, y=w602) -> (x*y=w604:sgl)
                  n190 = Multiply(x=w608, y=w602) -> (x*y=w603:sgl)
                  n191 = Add(x=w599, y=w606) -> (x+y=w592:sgl)
                  n192 = Add(x=w595, y=w605) -> (x+y=w589:sgl)
                  n193 = Add(x=w597, y=w604) -> (x+y=w591:sgl)
                  n194 = Add(x=w593, y=w603) -> (x+y=w590:sgl)
                }
                frame "Down to Up" {
                  n195 = Subtract(x=w621, y=w623) -> (x-y=w636:sgl)
                  n196 = Subtract(x=w626, y=w625) -> (x-y=w633:sgl)
                  n197 = Subtract(x=w620, y=w622) -> (x-y=w639:sgl)
                  n198 = Subtract(x=w627, y=w624) -> (x-y=w638:sgl)
                  n199 = Divide(x=w636, y=w628) -> (x/y=w635:sgl)
                  n200 = Divide(x=w633, y=w628) -> (x/y=w634:sgl)
                  n201 = Divide(x=w639, y=w628) -> (x/y=w640:sgl)
                  n202 = Divide(x=w638, y=w628) -> (x/y=w637:sgl)
                  n203 = Multiply(x=w635, y=w619) -> (x*y=w630:sgl)
                  n204 = Multiply(x=w634, y=w619) -> (x*y=w629:sgl)
                  n205 = Multiply(x=w640, y=w619) -> (x*y=w632:sgl)
                  n206 = Multiply(x=w637, y=w619) -> (x*y=w631:sgl)
                  n207 = Add(x=w623, y=w630) -> (x+y=w618:sgl)
                  n208 = Add(x=w625, y=w629) -> (x+y=w615:sgl)
                  n209 = Add(x=w622, y=w632) -> (x+y=w617:sgl)
                  n210 = Add(x=w624, y=w631) -> (x+y=w616:sgl)
                }
                frame "Right to Left" {
                  n211 = Subtract(x=w650, y=w649) -> (x-y=w662:sgl)
                  n212 = Subtract(x=w646, y=w645) -> (x-y=w659:sgl)
                  n213 = Subtract(x=w653, y=w652) -> (x-y=w665:sgl)
                  n214 = Subtract(x=w648, y=w647) -> (x-y=w664:sgl)
                  n215 = Divide(x=w662, y=w654) -> (x/y=w661:sgl)
                  n216 = Divide(x=w659, y=w654) -> (x/y=w660:sgl)
                  n217 = Divide(x=w665, y=w654) -> (x/y=w666:sgl)
                  n218 = Divide(x=w664, y=w654) -> (x/y=w663:sgl)
                  n219 = Multiply(x=w661, y=w651) -> (x*y=w656:sgl)
                  n220 = Multiply(x=w660, y=w651) -> (x*y=w655:sgl)
                  n221 = Multiply(x=w666, y=w651) -> (x*y=w658:sgl)
                  n222 = Multiply(x=w663, y=w651) -> (x*y=w657:sgl)
                  n223 = Add(x=w649, y=w656) -> (x+y=w643:sgl)
                  n224 = Add(x=w645, y=w655) -> (x+y=w641:sgl)
                  n225 = Add(x=w652, y=w658) -> (x+y=w644:sgl)
                  n226 = Add(x=w647, y=w657) -> (x+y=w642:sgl)
                }
              }
            }
          }
          n227 = Equal?(x=w464, y=w473) -> (x = y?=w471:bool)
          n228 = Or(x=w472, y=w471) -> ()  [unwired: 1 out]
          n229 = Bundle By Name(cluster=w459, "X"=w451, "Y"=w450) -> (w457:cluster{"X":i32, "Y":i32})
          n230 = Bundle By Name(cluster=w459, "X"=w448, "Y"=w449) -> (w458:cluster{"X":i32, "Y":i32})
          n231 = Bundle By Name(cluster=T19 {"Start X"=0, "Start Y"=0, "End X"=0, "End Y"=0} ("Line"), "Start X"=w451, "Start Y"=w450, "End X"=w448, "End Y"=w449) -> (w460:T19)
          n232 = Bundle By Name(cluster=T18 {"Point 1"={"x"=50.0, "y"=50.0}, "Point 2"={"x"=70.0, "y"=70.0}} ("Line Coordinates"), "Point 1"=w457, "Point 2"=w458) -> (w454:T18)
          n233 = call "Overlay Line with Arrows Simple.vi"("Color"=u32 16860, "error in"=w467, "Arrows"=cluster{"Start point":bool, "End point":bool} {"Start point"=FALSE, "End point"=TRUE}, "Line Coordinates"=w454, "Image In"=w470) -> ("error out"=w452:errorcluster, "Image Out"=w453:T2)  [unwired: 5 in]
          n234 = call "IMAQ Convert Line to ROI"("error in (no error)"=w452, "Line"=w460) -> ("error out"=w477:errorcluster, "ROI Descriptor"=w476:T22)  [unwired: 7 in]
          n235 = call "IMAQ Edge Tool 3"("Image"=w453, "Edge Options"=w482, "Optimized Mode"=FALSE, "ROI Descriptor"=w476, "Process"=w485, "error in (no error)"=w477) -> ("Image (duplicate)"=w486:T2, "Edge Information"=w489:T23[], "Gradient Values"=w480:dbl[], "error out"=w478:errorcluster)  [unwired: 5 in, 1 out]
          n236 = for {
            tunnel: w489 -> [w491] mode=indexing
            tunnel: [w490] -> w444 mode=indexing
            n237 = Unbundle By Name(w491) -> ("Location (Pixel)"=w490:cluster{"X":sgl, "Y":sgl})
          }
          n238 = call "IMAQ ROIProfile"("error in (no error)"=w478, "ROI Descriptor"=w476, "Image"=w453) -> ("error out"=w488:errorcluster, "ROI Graph"=w481:cluster{"x0":sgl, "dx":sgl, "Pixels Line":sgl[]})  [unwired: 1 in, 3 out]
          n239 = Index Array(array=w489, index=0) -> (element=w445:T23)
          n240 = Unbundle By Name(w445) -> ("Location (Pixel)"=w479:cluster{"X":sgl, "Y":sgl})
          n241 = call "Overlay Points with User Specified Size.vi"("Color"=u32 16711680, "error in"=w488, "Points"=w444, "Image In"=w486) -> ("error out"=w483:errorcluster, "Image Out"=w484:T2)  [unwired: 6 in]
        }
        "Line Profile" <- w329
        n242 = for {
          tunnel: w328 -> [w435] mode=indexing
          shift-right: [w434] -> w322
          shift-left: cluster{"X":sgl, "Y":sgl}[] [] -> [w433]
          n243 = Unbundle By Name(w435) -> ("X"=w439:sgl, "Y"=w438:sgl)
          n244 = Multiply(x=w439, y=w438) -> (x*y=w437:sgl)
          n245 = Not Equal To 0?(x=w437) -> (x != 0?=w436:bool)
          n246 = case shown="True" w436 {
            tunnel: w435 -> [_ w443]
            tunnel: [w440 w442] -> w434
            tunnel: w433 -> [w440 w441]
            frame False {
            }
            frame True {
              n247 = Build Array (concatenate)(w441, w443) -> (w442:cluster{"X":sgl, "Y":sgl}[])
            }
          }
        }
        n248 = Transpose 2D Array(2D array=w335) -> (transposed array=→"Gradient Information":dbl[][])
        n249 = case shown="3, 12, Default" w319 {
          tunnel: w327 -> [w342 w366]
          tunnel: w322 -> [w343 w351]
          tunnel: w321 -> [w340 w350]
          tunnel: [w341 w348] -> w320
          tunnel: [w339 w347] -> w314
          frame 7 {
            n250 = call "IMAQ Fit Ellipse 2"("error in (no error)"=w340, "Radial Points"=w343) -> ("error out"=w339:errorcluster, "Ellipse"=w344:T1)  [unwired: 4 in, 4 out]
            "Ellipse" <- w344
            n251 = Unbundle By Name(w344) -> ("Center"=w345:cluster{"X":sgl, "Y":sgl})
            n252 = Build Array(w345) -> (w346:cluster{"X":sgl, "Y":sgl}[])
            n253 = call "Overlay Points with User Specified Size.vi"("Points"=w346, "Image In"=w342) -> ("Image Out"=w341:T2)  [unwired: 8 in, 1 out]
          }
          frame 3, 12, Default {
            n254 = call "IMAQ Fit Line"("error in (no error)"=w350, "Pixel Radius"=sgl 10.0, "Points"=w351) -> ("error out"=w349:errorcluster, "Line Segment"=w364:T8)  [unwired: 3 in, 4 out]
            "Line Segment" <- w364
            n255 = Unbundle By Name(w364) -> ("Point 1"=w352:cluster{"X":sgl, "Y":sgl}, "Point 2"=w353:cluster{"X":sgl, "Y":sgl})
            n256 = Unbundle By Name(w352) -> ("X"=w362:sgl, "Y"=w360:sgl)
            n257 = Unbundle By Name(w353) -> ("X"=w361:sgl, "Y"=w359:sgl)
            n258 = call "IMAQ Overlay Line"("Color"=u32 16711680, "error in (no error)"=w349, "End Point"=w353, "Start Point"=w352, "Image"=w366) -> ("error out"=w347:errorcluster, "Image Out"=w348:T2)  [unwired: 5 in]
            n259 = Subtract(x=w362, y=w361) -> (x-y=w358:sgl)
            n260 = Subtract(x=w359, y=w360) -> (x-y=w357:sgl)
            n261 = Divide(x=w357, y=w358) -> (x/y=w356:sgl)
            n262 = Inverse Tangent(1:w356) -> (0:w355:sgl)
            n263 = expression code="(x/pi)*180.0" "radians to degrees"(w355) -> (→"degrees":sgl)
          }
        }
        "error out" <- w314
      }
    }
    "Image" <- w291
  }
